vi "Switch Configuration - Initialize Switch Configuration.vi"(8 "error in (no error)":errorcluster, 10 "Switch Config UI Data in":T2 {"Switch Config Page Item Ref" format="%.0x"}, 11 "Item Ref in":T1 format="%.0x") -> (0 "error out":errorcluster, 2 "Switch Config UI Data out":T2 {"Switch Config Page Item Ref" format="%.0x"})   [LabVIEW 2015, in "DMM-SWITCH-ScanList System Explorer.lvlib"]
doc: "Read saved properties and update UI controls and indicators values and properties. Some extra processing an filtering is used to fill in some controls and indicators."
uses:
  DMM-SWITCH-ScanList System Explorer.lvlib
  Configuration Controls/Switch Config VI UI Data.ctl
  Configuration Controls/Switch Config VI UI Ctrl Values.ctl
  Configuration Controls/Switch Config VI UI Ctrl References.ctl
  <instrlib>/niSwitch/niSwitch.LLB/niSwitch Topologies.ctl
  <vilib>/NI Veristand/Custom Device API/Custom Device Item Ref.ctl
  Shared/Constants.vi
  <vilib>/NI Veristand/Custom Device API/Get Item Property (String).vi
  <vilib>/NI Veristand/Custom Device API/Get Item Property (String Array).vi
  <vilib>/NI Veristand/Custom Device API/Get Item Property (Boolean).vi
  <vilib>/NI Veristand/Custom Device API/Custom Device API.lvlib
  Shared/DMM-SWITCH-ScanList Shared.lvlib
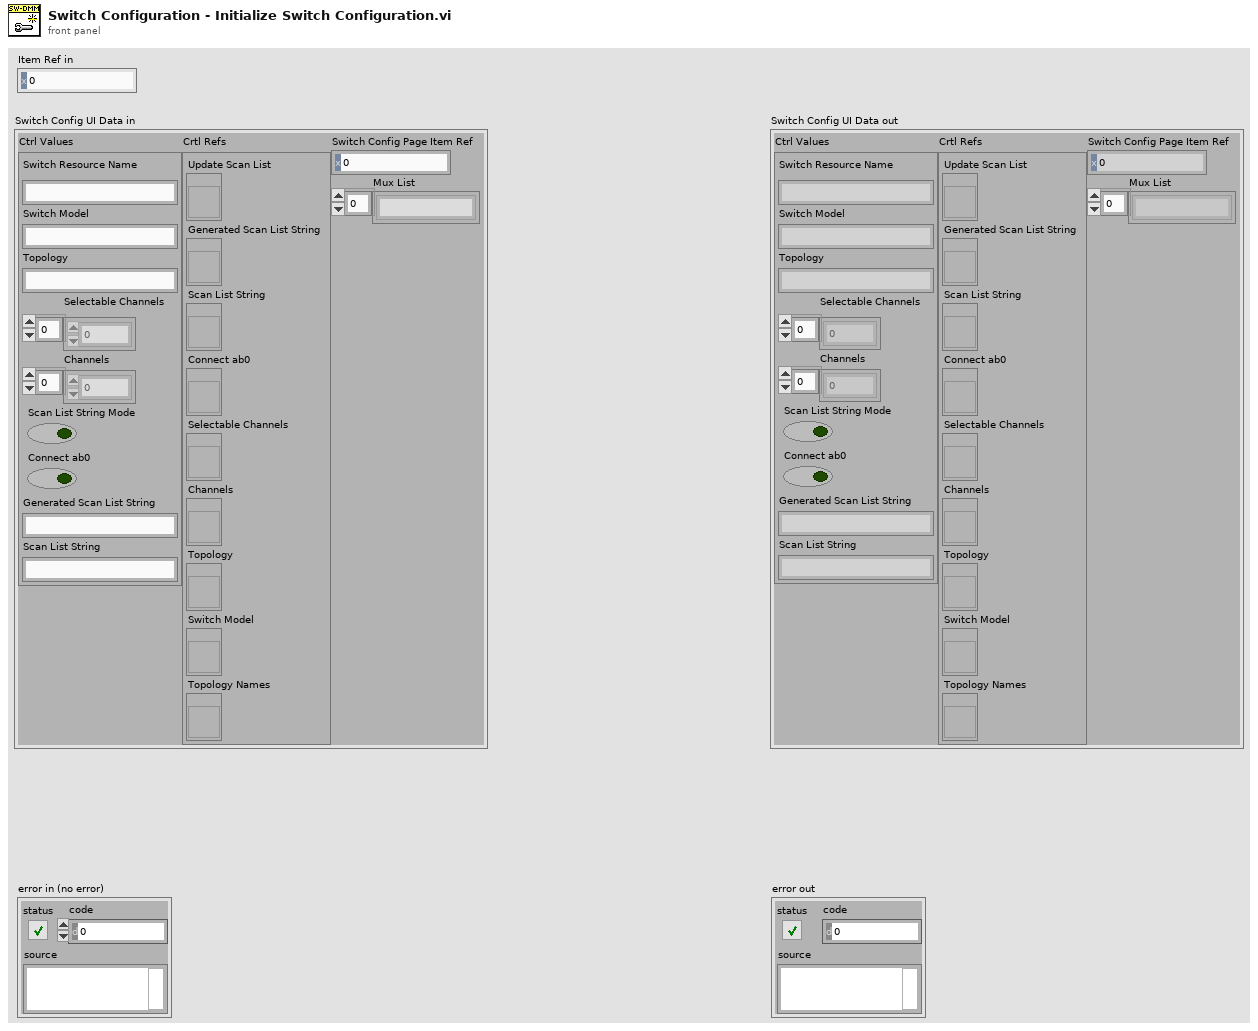
[diagram p1: front panel]
types:
  T1 = typedef "Custom Device API.lvlib/Custom Device Item Ref.ctl" = u64
  T2 = typedef "DMM-SWITCH-ScanList System Explorer.lvlib/Switch Config VI UI Data.ctl" = cluster{"Ctrl Values":T3, "Crtl Refs":T4, "Switch Config Page Item Ref":T1, "Mux List":string[]}
  T3 = typedef "DMM-SWITCH-ScanList System Explorer.lvlib/Switch Config VI UI Ctrl Values.ctl" = cluster{"Switch Resource Name":string, "Switch Model":string, "Topology":string, "Selectable Channels":i32[], "Channels":i32[], "Scan List String Mode":bool, "Connect ab0":bool, "Generated Scan List String":string, "Scan List String":string}
  T4 = typedef "DMM-SWITCH-ScanList System Explorer.lvlib/Switch Config VI UI Ctrl References.ctl" = cluster{"Update Scan List":refnum<vi>, "Generated Scan List String":refnum<vi>, "Scan List String":refnum<vi>, "Connect ab0":refnum<vi>, "Selectable Channels":refnum<vi>, "Channels":refnum<vi>, "Topology":refnum<vi>, "Switch Model":refnum<vi>, "Topology Names":refnum<vi>}
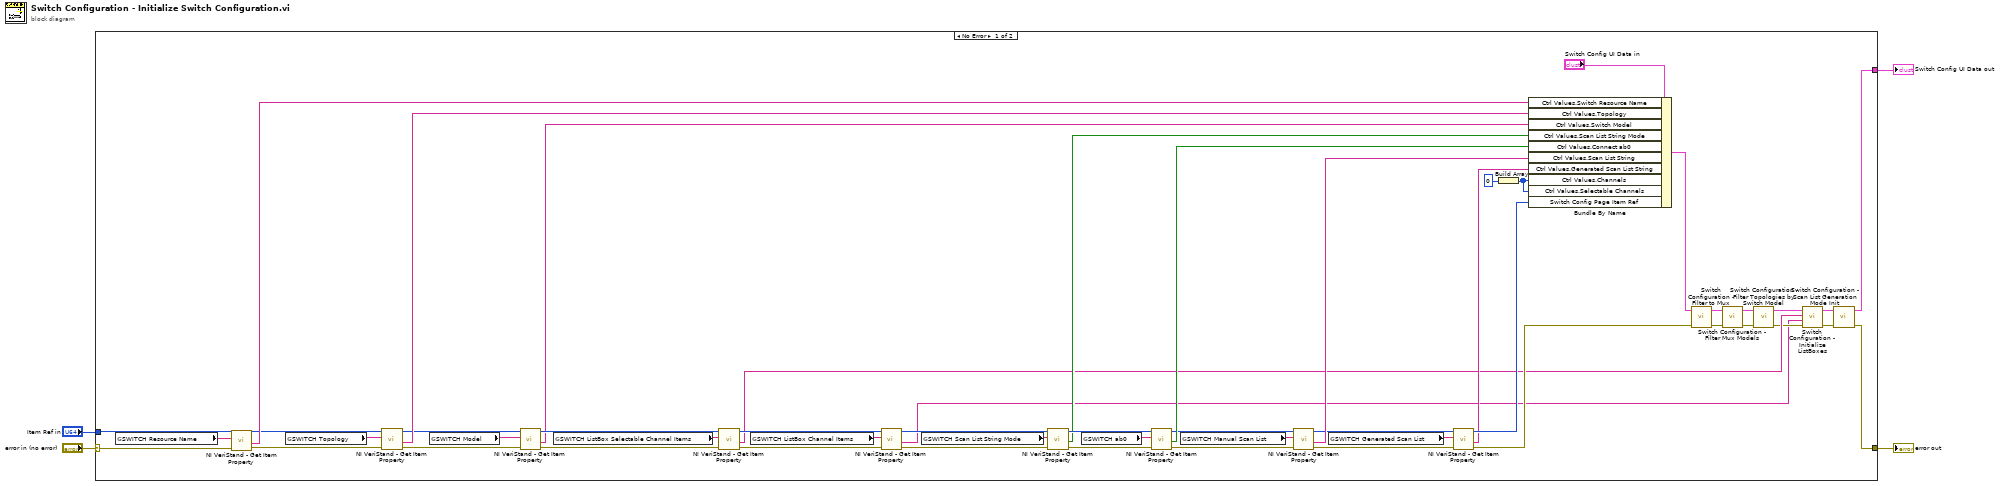
[diagram p0: block diagram]
diagram:
  n1 = case shown="No Error" "error in (no error)" {
    selector: "error in (no error)" -> [w35 w57]
    tunnel: [w14 _] -> w4
    tunnel: [w56 w57] -> w3
    tunnel: "Item Ref in" -> [w39 _]
    frame No Error {
      n2 = global read "Constants.vi" "SWITCH Resource Name"() -> (w13:string)
      n3 = call-poly <vilib>:"NI VeriStand - Get Item Property.vi"("error in (no error)"=w35, "Property Name"=w13, "Item Ref in"=w39) -> ("error out"=w37:errorcluster, "Value"=w50:string, "Item Ref out"=w38:T1)  [unwired: 5 in, 1 out]
      n4 = global read "Constants.vi" "SWITCH Topology"() -> (w12:string)
      n5 = call-poly <vilib>:"NI VeriStand - Get Item Property.vi"("error in (no error)"=w37, "Property Name"=w12, "Item Ref in"=w38) -> ("error out"=w29:errorcluster, "Value"=w51:string, "Item Ref out"=w26:T1)  [unwired: 5 in, 1 out]
      n6 = global read "Constants.vi" "SWITCH Model"() -> (w11:string)
      n7 = call-poly <vilib>:"NI VeriStand - Get Item Property.vi"("error in (no error)"=w29, "Property Name"=w11, "Item Ref in"=w26) -> ("error out"=w28:errorcluster, "Value"=w25:string, "Item Ref out"=w27:T1)  [unwired: 5 in, 1 out]
      n8 = global read "Constants.vi" "SWITCH ListBox Selectable Channel Items"() -> (w10:string)
      n9 = call-poly <vilib>:"NI VeriStand - Get Item Property.vi"("error in (no error)"=w28, "Property Name"=w10, "Item Ref in"=w27) -> ("error out"=w40:errorcluster, "Value"=w18:string[], "Item Ref out"=w41:T1)  [unwired: 5 in, 1 out]
      n10 = global read "Constants.vi" "SWITCH ListBox Channel Items"() -> (w9:string)
      n11 = call-poly <vilib>:"NI VeriStand - Get Item Property.vi"("error in (no error)"=w40, "Property Name"=w9, "Item Ref in"=w41) -> ("error out"=w47:errorcluster, "Value"=w16:string[], "Item Ref out"=w45:T1)  [unwired: 5 in, 1 out]
      n12 = global read "Constants.vi" "SWITCH Scan List String Mode"() -> (w8:string)
      n13 = call-poly <vilib>:"NI VeriStand - Get Item Property.vi"("error in (no error)"=w47, "Property Name"=w8, "Item Ref in"=w45) -> ("error out"=w44:errorcluster, "Value"=w23:bool, "Item Ref out"=w46:T1)  [unwired: 5 in, 1 out]
      n14 = global read "Constants.vi" "SWITCH ab0"() -> (w7:string)
      n15 = call-poly <vilib>:"NI VeriStand - Get Item Property.vi"("error in (no error)"=w44, "Property Name"=w7, "Item Ref in"=w46) -> ("error out"=w42:errorcluster, "Value"=w52:bool, "Item Ref out"=w43:T1)  [unwired: 5 in, 1 out]
      n16 = global read "Constants.vi" "SWITCH Manual Scan List"() -> (w6:string)
      n17 = call-poly <vilib>:"NI VeriStand - Get Item Property.vi"("error in (no error)"=w42, "Property Name"=w6, "Item Ref in"=w43) -> ("error out"=w34:errorcluster, "Value"=w53:string, "Item Ref out"=w32:T1)  [unwired: 5 in, 1 out]
      n18 = global read "Constants.vi" "SWITCH Generated Scan List"() -> (w5:string)
      n19 = call-poly <vilib>:"NI VeriStand - Get Item Property.vi"("error in (no error)"=w34, "Property Name"=w5, "Item Ref in"=w32) -> ("error out"=w33:errorcluster, "Value"=w30:string, "Item Ref out"=w31:T1)  [unwired: 5 in, 1 out]
      n20 = Build Array(0) -> (w55:i32[])
      n21 = Bundle By Name(cluster="Switch Config UI Data in", "Ctrl Values.Switch Resource Name"=w50, "Ctrl Values.Topology"=w51, "Ctrl Values.Switch Model"=w25, "Ctrl Values.Scan List String Mode"=w23, "Ctrl Values.Connect ab0"=w52, "Ctrl Values.Scan List String"=w53, "Ctrl Values.Generated Scan List String"=w30, "Ctrl Values.Channels"=w55, "Ctrl Values.Selectable Channels"=w55, "Switch Config Page Item Ref"=w31) -> (w22:T2)
      n22 = call "Switch Configuration - Filter to Mux.vi"("error in (no error)"=w33, "Switch Config UI Data In"=w22) -> ("error out"=w36:errorcluster, "Switch Config UI Data Out"=w21:T2)  [unwired: 8 in]
      n23 = call "Switch Configuration - Filter Mux Models.vi"("error in (no error)"=w36, "Switch Config UI Data In"=w21) -> ("error out"=w48:errorcluster, "Switch Config UI Data Out"=w20:T2)  [unwired: 7 in, 1 out]
      n24 = call "Switch Configuration - Filter Topologies by Switch Model.vi"("error in (no error)"=w48, "Switch Config UI Data In"=w20) -> ("error out"=w17:errorcluster, "Switch Config UI Data Out"=w19:T2)  [unwired: 7 in, 1 out]
      n25 = call "Switch Configuration - Initialize ListBoxes.vi"("error in (no error)"=w17, "Channels ListBox Items"=w16, "Selectable Channels ListBox Items"=w18, "Switch Config UI Data In"=w19) -> ("error out"=w24:errorcluster, "Switch Config UI Data Out"=w15:T2)  [unwired: 6 in]
      n26 = call "Switch Configuration - Scan List Generation Mode Init.vi"("error in (no error)"=w24, "Switch Config UI Data In"=w15) -> ("error out"=w56:errorcluster, "Switch Config UI Data Out"=w14:T2)  [unwired: 8 in]
    }
    frame Error {
    }
  }
  "Switch Config UI Data out" <- w4
  "error out" <- w3
